vi "SCMP - Externally Triggered Image Acquisition - v4.vi"(0 "FPS":dbl=10.0 format="%.1g", 1 "LCVR Voltages":dbl[][](array[numeric]), 2 "Mod/Seq":bool, 5 "Cycles":i32=1 min=1 max=30 step=1, 7 "Save to FITS?":bool=TRUE, 9 "Headers In":T12[](array[typedef])=[{"Wavelength (nm)"=530.15, "Exposure (s)"=0.05, "Tuning Delay (ms)"=1000.0, "Beam Type (-1/1)"=1.0, "Tuning Voltages"=[1.111, 2.222, 3.333, 4.444], "Observer"="observer", "Light Shapping Diffuser"=enum."In Beam", "Comment"="", "Data Type"=9, "Mod Cycles"=0, "SCD Calibration Optics"=enum."1 - Polarizer @0, I+Q", "SCD Emission Line Filter"=enum."1-557.6nm", "Cookbook"="", "COMP-S Calibration Wheel"=enum."Dark", "COMP-S Andover Filter Wheel"=enum."530.3nm/HWB 0.34nm (Fe XIV)", "FOV Rotation (deg)"=66.0, "Objective Lens Position (mm)"=0.0, "Occulter size"=0.0, "Time End"=timestamp(3382374145.421875 s since 1904-01-01), "Acc Exposure (s)"=0.0, "Time Stamp Array"=[], "Camera Serial Number"=[], "Camera Temp"=[], "Camera PI (mm)"=[], "Time Start"=timestamp(3382374145.421875 s since 1904-01-01), "Peripherals"={"ILX controler"=FALSE, "Zone temperatures"=FALSE, "Andor"=FALSE, "Andor 2"=FALSE, "PI Stages"=FALSE, "AISAS mechanisms"=FALSE, "AISAS Mech.lvclass"=refnum, "Zone temp ref"=variant, "FWs"=FALSE}, "FITS paths"=[], "Cameras"=enum."Andor", "load preset cbk"=FALSE, "periodic check count"=0, "COMP-S Calibration Wheel 2"=enum."Dark", "Calib"=enum."Dark", "Abso Aperture"=40.0, "Nominal Aperture"=196.0}] {"Nominal Aperture" format="%.1f"; "Abso Aperture" format="%.1f"; "Camera PI (mm)" format="%_3g"; "Acc Exposure (s)" format="%^.3g"; "Occulter size" format="%.2f"; "Objective Lens Position (mm)" min=70.0 max=152.0 format="%.2f"; "FOV Rotation (deg)" format="%.1f"; "Data Type" items=["LIVE", "DARK", "FLAT", "CALI", "OBSE", "ABSO", "AURE", "TARG", "OBJE", "HOLE", "OREX", "THRO", "CHIP"]; "Exposure (s)" format="%^.3g"; "Wavelength (nm)" format="%_6g"}, 11 "error in":errorcluster, 12 "Andor Neo":T13[](array[typedef]) {"Exposure (s)" format="%^.3g"; "Time at Synch" format="%<%H:%M:%S>T"; "Interframe Time" format="%#_3g"; "Frame Readout Time" format="%_3g"; "Row Readout Time" format="%_3g"}) -> (3 "FITS Path Out":path, 6 "Image":u32[][](array[numeric]), 8 "Camera R Image":u32[][](graph), 10 "Headers Out":T2[](array[typedef]) {"Nominal Aperture" format="%.1f"; "Abso Aperture" format="%.1f"; "Camera PI (mm)" format="%_3g"; "Acc Exposure (s)" format="%^.3g"; "Occulter size" format="%.2f"; "Objective Lens Position (mm)" min=70.0 max=152.0 format="%.2f"; "FOV Rotation (deg)" format="%.1f"; "Exposure (s)" format="%^.3g"; "Wavelength (nm)" format="%_6g"}, 13 "FITS Path Out 2":path, 14 "Break":bool, 15 "error out":errorcluster)   [LabVIEW 2014]
doc: "The LL Sequence VI acquires a sequence of images and displays them in an array of image controls using the low-level acquisition VIs. A sequence is appropriate for applications that process multiple images. You can configure a sequence to acquire every frame or to skip a variable number of frames between each image.\n\nTop Level Code Overview\n1) Initialize Camera (Global Shutter, High Well, Low Noise, exposure time, etc.)\n2) Create a buffer set equal in size to the # of trigger pulses (e.g. 100) which is the same as the # of expected images \n3) Start the camera acquisition THEN start the DAQmx task (use merge error cluster to gurantee this)"
uses:
  Camera/Andor Neo Info.ctl
  Controls/run cbk timeout.ctl
  <vilib>/Waveform/WDTOps.llb/WDT Waveform Duration DBL.vi
  <vilib>/DAQmx/write.llb/DAQmx Write (Analog 1D Wfm NChan NSamp).vi
  <vilib>/DAQmx/create/channels.llb/DAQmx Create Channel (AO-Voltage-Basic).vi
  <vilib>/DAQmx/configure/timing.llb/DAQmx Timing (Use Waveform).vi
  Controls/Global demo.vi
  Controls/beaning.ctl
  Controls/SCD - Calibration Optics Filter Wheel.ctl
  AISAS/Controls/Diffuser.ctl
  Controls/SCD - FITS Cluster.ctl
  Controls/SCD - EDT - Emission Line Filter Wheel.ctl
  Controls/CoMP-S Controls/Polarization Optics Filter Wheel.ctl
  Controls/CoMP-S Controls/Emission Line Filter Wheel.ctl
  AISAS/Controls/focus.ctl
  AISAS/Mech/AISAS Mech.lvclass
  Controls/peripherals.ctl
  Controls/Cameras select.ctl
  Controls/FITS Data type.ctl
panel:
  out "error dequeue RAM":errorcluster
  out "mod cycles *4":i32=1
  out "error cam dequeue & queue RAM":errorcluster
  out "error dequeue 2":errorcluster
  in  "count 2":i32
  in  "Tab Control":T1(tab)
  out "Camera T Image":u32[][](graph)
  out "# elements in RAM queue":i32
  out "Image Acq (s)":dbl(slide)=4151.832132564842
  out "Image display & SSD Saving":i32(slide) scale=0.0..1.0
  in  "user break":bool
  out "Camera T Image wide":u32[][](graph)
  out "# images to acquire":i32
  out "Image Acquisition Started":bool
  out "PixelData [U16]":u16[](array[numeric])
  out "ByteData [U8]":u8[](array[numeric])
  in  "image pointers":u64[](array[numeric])
  in  "imageNo":i32
  in  "count":i32
  out "# wavelengths":i32=1
  out "Exposure Get (s)":dbl=0.09 format="%_3p"
  out "# elements in queue":i32
  out "Image Cam":u32[][](graph)
  out "# buffer":i32
  in  "image pointers 2":u64[](array[numeric])
  in  "imageNo 2":i32
  out "# elements in queue 2":i32
  out "# buffer 2":i32
  out "Image transfering":u32(slide) scale=0.0..4.0
  out "Acquisition Estimate (s)":dbl format="%0.2f"
  out "Image Acq":i32(slide) scale=0.0..4.0
  out "Time Start":timestamp=timestamp(3382374145.421875 s since 1904-01-01) format="%<%H:%M:%S%3u\n%x>T"
  out "Time stamp arr":timestamp[](array[timestamp]) format="%<%H:%M:%S%3u>T"
  out "COMP Waveforms":waveform(dbl)[](graph)
  out "SCD Waveforms":waveform(dbl)[](graph)
  out "Time stamp arr 2":timestamp[](array[timestamp]) format="%<%H:%M:%S%3u>T"
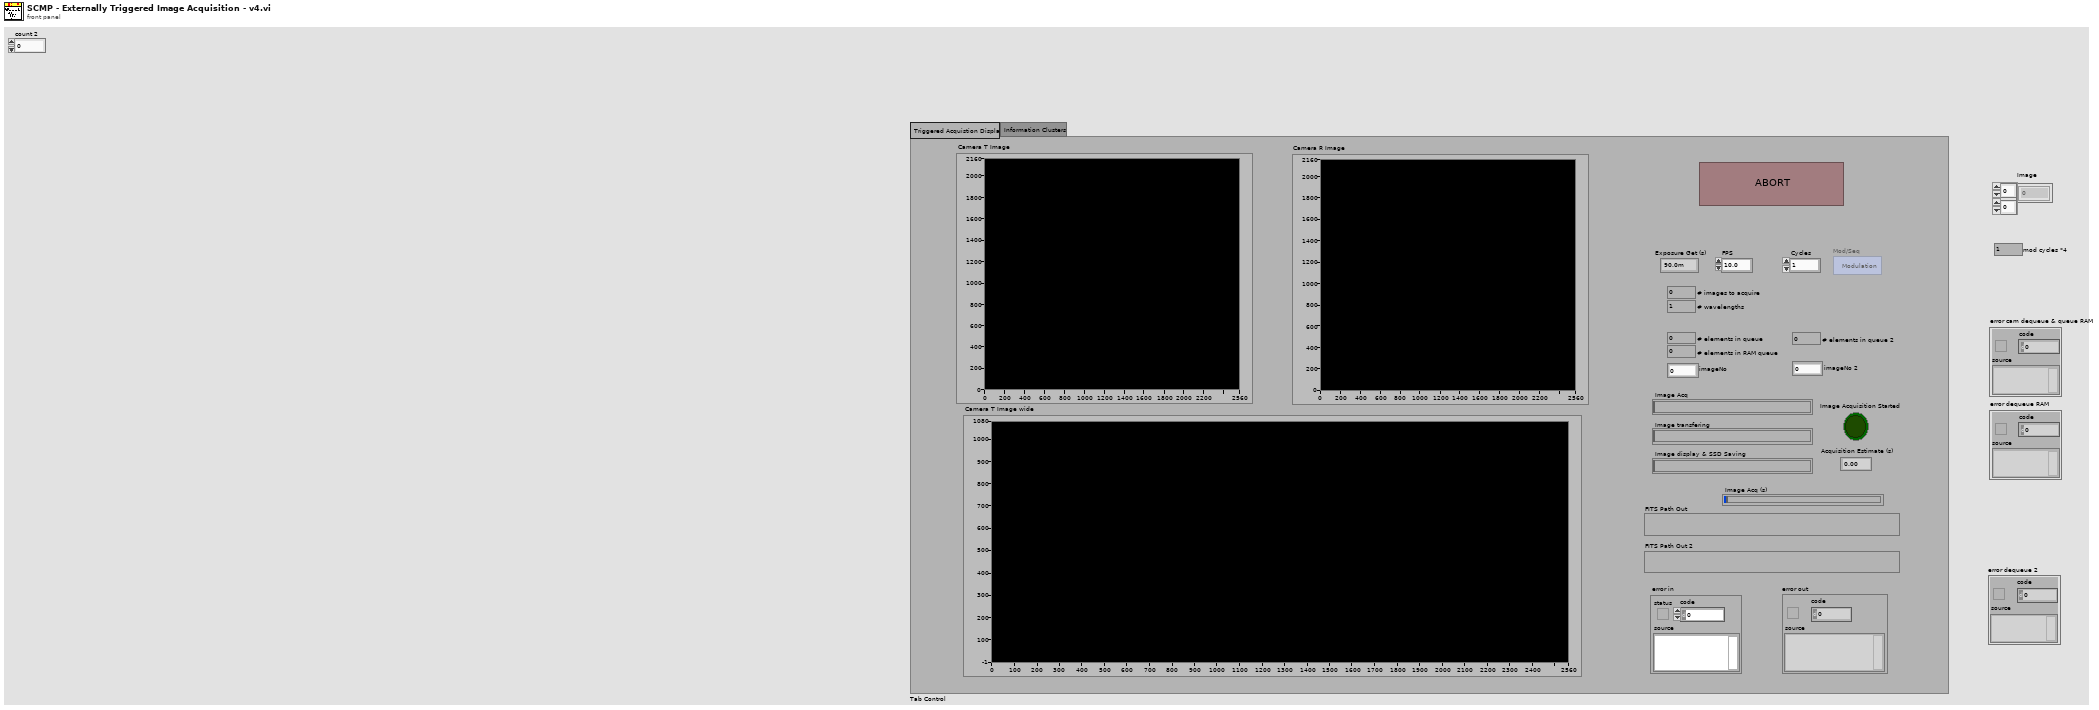
[diagram p1: front panel]
types:
  T1 = enum32{"Triggered Acquistion Display", "Information Clusters"}
  T2 = typedef "SCD - FITS Cluster.ctl" = cluster{"Wavelength (nm)":dbl, "Exposure (s)":dbl, "Tuning Delay (ms)":dbl, "Beam Type (-1/1)":dbl, "Tuning Voltages":dbl[], "Observer":string, "Light Shapping Diffuser":T3, "Comment":string, "Data Type":T4, "Mod Cycles":u16, "SCD Calibration Optics":T5, "SCD Emission Line Filter":T6, "Cookbook":string, "COMP-S Calibration Wheel":T7, "COMP-S Andover Filter Wheel":T8, "FOV Rotation (deg)":dbl, "Objective Lens Position (mm)":T9, "Occulter size":dbl, "Time End":timestamp, "Acc Exposure (s)":dbl, "Time Stamp Array":timestamp[], "Camera Serial Number":string[], "Camera Temp":dbl[], "Camera PI (mm)":dbl[], "Time Start":timestamp, "Peripherals":T10, "FITS paths":path[], "Cameras":T11, "load preset cbk":bool, "periodic check count":i32, "COMP-S Calibration Wheel 2":T7, "Calib":enum16{"Dark", "Flat"}, "Abso Aperture":dbl, "Nominal Aperture":dbl, "Pointer IP":string}
  T3 = typedef "Diffuser.ctl" = enum16{"Out of Beam", "In Beam"}
  T4 = typedef "FITS Data type.ctl" = enum16{"LIVE", "DARK", "FLAT", "CALI", "OBSE", "ABSO", "AURE", "TARG", "OBJE", "HOLE", "OREX", "THRO", "CHIP"}
  T5 = typedef "SCD - Calibration Optics Filter Wheel.ctl" = enum16{"1 - Polarizer @0, I+Q", "2 - Polarizer @90, I-Q", "3 - Polarizer @45, I+U", "4 - Polarizer @135, I-U", "5 - Polarizer @0, Retarder @45, I+V", "6 - Polarizer @0, Retarder @135, I-V", "7 - Dark", "8 - Clear", "9 - N/A"}
  T6 = typedef "SCD - EDT - Emission Line Filter Wheel.ctl" = enum16{"1-557.6nm", "2-587.6nm", "3-589.6nm", "4-630.2nm", "5-656.4nm", "6-849.8nm", "7-854.2nm", "8-866.2nm", "9-1083.0nm"}
  T7 = typedef "Polarization Optics Filter Wheel.ctl" = enum16{"Dark", "Clear", "Exchange Lens", "Polarizer @0, I+Q", "Polarizer @90, I-Q", "Polarizer @45, I+U", "Polarizer @135, I-U", "Polarizer @0, Retarder @45, I+V", "Polarizer @0, Retarder @135, I-V"}
  T8 = typedef "Emission Line Filter Wheel.ctl" = enum16{"530.3nm/HWB 0.34nm (Fe XIV)", "587.6nm/HBW 0.44nm (He I D3)", "637.5nm/HBW 0.53nm (Fe X)", "656.3nm/HBW 0.57nm (H-Alpha)", "789.2nm/HBW 0.85nm (Fe XI)", "854.2nm/HBW 1.01nm (Ca I)", "1074.7nm/HBW 2.34nm (Fe XIII)", "1079.8nm/HBW 1.64nm (Fe XIII)", "1083.0nm/HBW 1.66nm (He I)"}
  T9 = typedef "focus.ctl" = dbl
  T10 = typedef "peripherals.ctl" = cluster{"ILX controler":bool, "Zone temperatures":bool, "Andor":bool, "Andor 2":bool, "PI Stages":bool, "AISAS mechanisms":bool, "AISAS Mech.lvclass":refnum<class "AISAS Mech.lvclass">, "Zone temp ref":variant, "FWs":bool}
  T11 = typedef "Cameras select.ctl" = enum16{"Andor", "GDR"}
  T12 = typedef "SCD - FITS Cluster.ctl" = cluster{"Wavelength (nm)":dbl, "Exposure (s)":dbl, "Tuning Delay (ms)":dbl, "Beam Type (-1/1)":dbl, "Tuning Voltages":dbl[], "Observer":string, "Light Shapping Diffuser":T3, "Comment":string, "Data Type":u16, "Mod Cycles":u16, "SCD Calibration Optics":T5, "SCD Emission Line Filter":T6, "Cookbook":string, "COMP-S Calibration Wheel":T7, "COMP-S Andover Filter Wheel":T8, "FOV Rotation (deg)":dbl, "Objective Lens Position (mm)":T9, "Occulter size":dbl, "Time End":timestamp, "Acc Exposure (s)":dbl, "Time Stamp Array":timestamp[], "Camera Serial Number":string[], "Camera Temp":dbl[], "Camera PI (mm)":dbl[], "Time Start":timestamp, "Peripherals":T10, "FITS paths":path[], "Cameras":T11, "load preset cbk":bool, "periodic check count":i32, "COMP-S Calibration Wheel 2":T7, "Calib":enum16{"Dark", "Flat"}, "Abso Aperture":dbl, "Nominal Aperture":dbl}
  T13 = typedef "Andor Neo Info.ctl" = cluster{"Handle":i32, "Pixel Encoding":string, "AOI Width":i32, "AOI Height":i32, "AOI Stride":i32, "Row Readout Time":dbl, "Frame Readout Time":dbl, "Interframe Time":dbl, "Semaphore":T14, "SerialNumber":string, "Camera Model":string, "Controller ID":string, "Firmware Version":string, "Shutter":string, "BDiv":u8, "Time at Synch":timestamp, "Idx":i32, "PreAmp":string, "Binning":T15, "PixelReadoutRate":string, "Exposure (s)":dbl, "Image Bytes":i64, "Image Pixels":i64, "SpuriousNoiseFilter":bool, "Overlap":bool, "CycleMode":string}
  T14 = typedef "Semaphore RefNum" = refnum<k1>
  T15 = typedef "beaning.ctl" = enum16{"1x1", "2x2", "3x3", "4x4", "8x8"}
  T16 = enum8{"Enabled", "Disabled", "Disabled and Grayed Out"}
  T17 = typedef "run cbk timeout.ctl" = i32
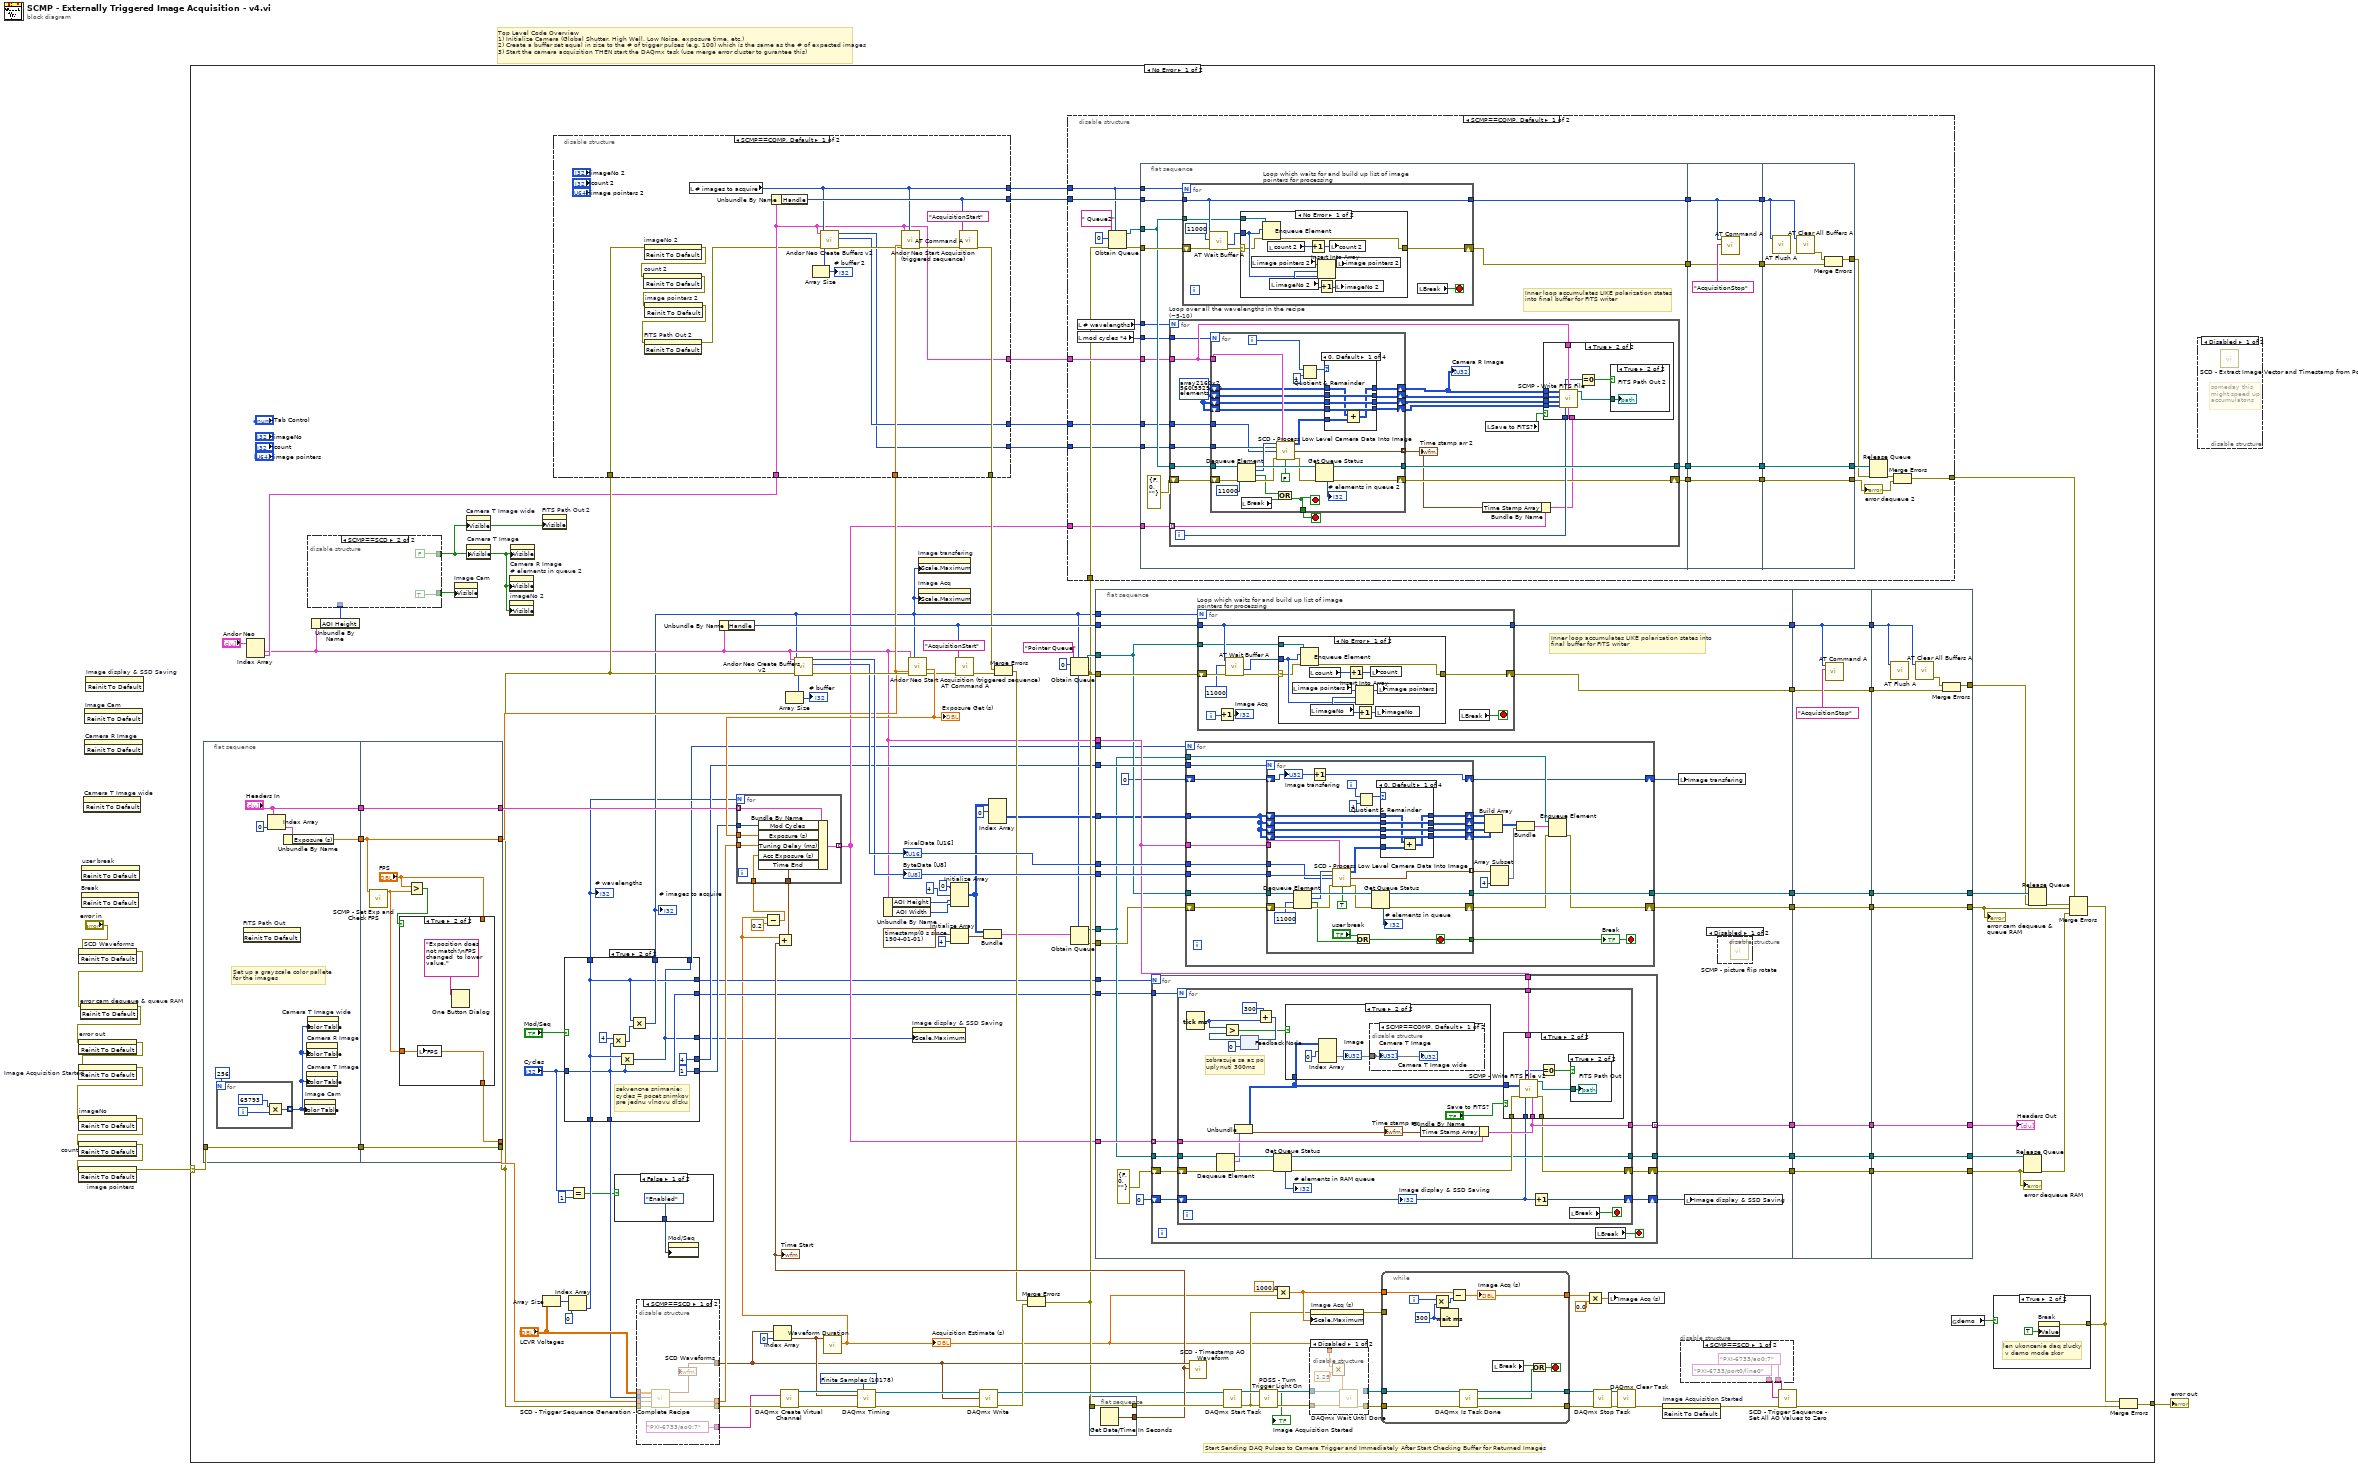
[diagram p0: block diagram]
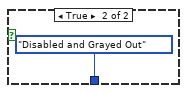
[diagram p3: hidden frame]
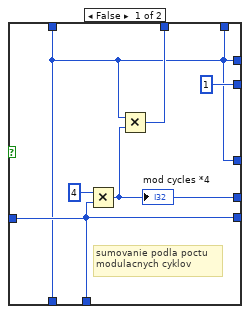
[diagram p6: hidden frame]
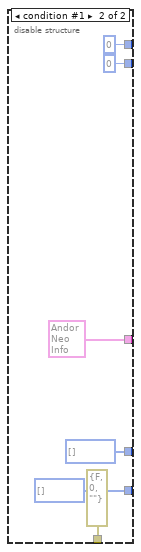
[diagram p7: hidden frame]
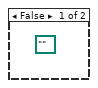
[diagram p8: hidden frame]
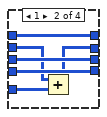
[diagram p10: hidden frame]
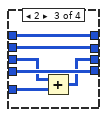
[diagram p11: hidden frame]
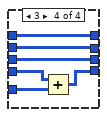
[diagram p12: hidden frame]
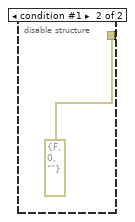
[diagram p14: hidden frame]
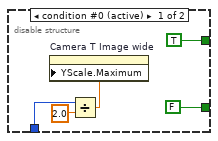
[diagram p16: hidden frame]
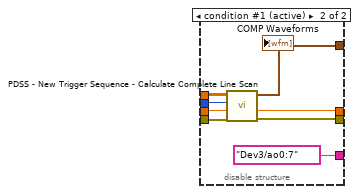
[diagram p17: hidden frame]
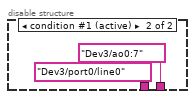
[diagram p18: hidden frame]
diagram:
  # "Top Level Code Overview\n1) Initialize Camera (Global Shutter, High Well, Low Noise, exposure time, etc.)\n2) Create a buffer set equal in size to the # of trigger pulses (e.g. 100) which is the same as the # of expected images \n3) Start the camera acquisition THEN start the DAQmx task (use merge error cluster to gurantee this)"
  n1 = invoke on="SCD Waveforms" class="WFGraph (strict)" method="Reinit To Default"(error in="error in") -> (error out=w3:errorcluster)  [unwired: 2 in, 2 out]
  n2 = invoke on="error cam dequeue & queue RAM" class="Clust (strict)" method="Reinit To Default"(error in=w3) -> (error out=w2:errorcluster)  [unwired: 2 in, 2 out]
  n3 = invoke on="error out" class="Clust (strict)" method="Reinit To Default"(error in=w2) -> (error out=w8:errorcluster)  [unwired: 2 in, 2 out]
  n4 = invoke on="Image Acquisition Started" class="Bool (strict)" method="Reinit To Default"(error in=w8) -> (error out=w4:errorcluster)  [unwired: 2 in, 2 out]
  n5 = invoke on="imageNo" class="DigNum (strict)" method="Reinit To Default"(error in=w4) -> (error out=w7:errorcluster)  [unwired: 2 in, 2 out]
  n6 = invoke on="count" class="DigNum (strict)" method="Reinit To Default"(error in=w7) -> (error out=w6:errorcluster)  [unwired: 2 in, 2 out]
  n7 = invoke on="image pointers" class="Arr (strict)" method="Reinit To Default"(error in=w6) -> (error out=w5:errorcluster)  [unwired: 2 in, 2 out]
  n8 = invoke on="Break" class="Bool (strict)" method="Reinit To Default"() -> ()  [unwired: 3 in, 3 out]
  n9 = invoke on="user break" class="Bool (strict)" method="Reinit To Default"() -> ()  [unwired: 3 in, 3 out]
  n10 = invoke on="Camera T Image wide" class="IntGraph (strict)" method="Reinit To Default"() -> ()  [unwired: 3 in, 3 out]
  n11 = invoke on="Image Cam" class="IntGraph (strict)" method="Reinit To Default"() -> ()  [unwired: 3 in, 3 out]
  n12 = invoke on="Camera R Image" class="IntGraph (strict)" method="Reinit To Default"() -> ()  [unwired: 3 in, 3 out]
  n13 = invoke on="Image display & SSD Saving" class="Slide (strict)" method="Reinit To Default"() -> ()  [unwired: 3 in, 3 out]
  n14 = case shown="No Error" w5 {
    selector: w5 -> [w92 w610]
    tunnel: [w120 w610] -> w9
    frame No Error {
      w143 = 10178 items=["Finite Samples"=10178, "Continuous Samples"=10123] ("sample mode")
      # "Start Sending DAQ Pulses to Camera Trigger and Immediately After Start Checking Buffer for Returned Images"
      n15 = flat-sequence {
        tunnel: w92 -> [w365]
        tunnel: [w365] -> w84
        tunnel: ["Headers In"] -> w82
        tunnel: [w361] -> w81
        tunnel: [w376] -> w63
        tunnel: w84 -> [w376]
        tunnel: [w375] -> w83
        tunnel: w82 -> [w375]
        tunnel: [w370] -> w73
        tunnel: w81 -> [w370]
        tunnel: [w373] -> w80
        frame #0 {
          # "Set up a grayscale color pallete for the images"
          n16 = for {
            N: 256 -> [_]
            tunnel: [w368] -> w360 mode=indexing
            i -> [w369]
            n17 = Multiply(x=65793, y=w369) -> (x*y=w368:i32)
          }
          n18 = invoke on="FITS Path Out" class="Path" method="Reinit To Default"() -> ()  [unwired: 3 in, 3 out]
          n19 = Index Array(array="Headers In", index=0) -> (element=w363:T12)
          n20 = Unbundle By Name(w363) -> ("Exposure (s)"=w361:dbl)
          n21 = property on="Image Cam" class="IntGraph (strict)"("Color Table"=w360) -> ()  [unwired: 2 in, 2 out]
          n22 = property on="Camera R Image" class="IntGraph (strict)"("Color Table"=w360) -> ()  [unwired: 2 in, 2 out]
          n23 = property on="Camera T Image" class="IntGraph (strict)"("Color Table"=w360) -> ()  [unwired: 2 in, 2 out]
          n24 = property on="Camera T Image wide" class="IntGraph (strict)"("Color Table"=w360) -> ()  [unwired: 2 in, 2 out]
        }
        frame #1 {
          n25 = call "SCMP - Set Exp and Check FPS.vi"("Exposure [s]"=w370) -> ("FPS"=w371:dbl)  [unwired: 9 in, 1 out]
          n26 = Greater?(x="FPS", y=w371) -> (0:w374:bool)
          n27 = case shown="True" w374 {
            tunnel: [w377 w378] -> w373
            tunnel: "FPS" -> [w377 _]
            tunnel: w371 -> [_ w378]
            frame False {
            }
            frame True {
              n28 = local write "FPS"(w378) -> ()
              n29 = One Button Dialog(message="Exposition does not match!\nFPS changed  to lower value.") -> ()  [unwired: 1 in, 1 out]
            }
          }
        }
      }
      n30 = Index Array(array="Andor Neo") -> (element #1=w55:T13, element #2=w60:T13)  [unwired: 2 in]
      n31 = Unbundle By Name(w55) -> ("AOI Height"=w99:i32)
      n32 = disable-structure shown="SCMP==SCD" {
        disable-tunnel: w99 -> [w383 _]
        disable-tunnel: [TRUE ("Visible") FALSE ("Visible")] -> w10
        disable-tunnel: [FALSE ("Visible") TRUE ("Visible")] -> w98
        frame condition #0 (active) {
          n33 = Divide(x=w383, y=2.0) -> (x/y=w384:dbl)
          n34 = property on="Camera T Image wide" class="IntGraph (strict)"("YScale.Maximum"=w384) -> ()  [unwired: 2 in, 2 out]
        }
        frame condition #1 {
        }
      }
      n35 = property on="Image Cam" class="IntGraph (strict)"("Visible"=w98) -> ()  [unwired: 2 in, 2 out]
      n36 = property on="Camera T Image wide" class="IntGraph (strict)"("Visible"=w10) -> ()  [unwired: 2 in, 2 out]
      n37 = property on="Camera T Image" class="IntGraph (strict)"("Visible"=w10) -> ()  [unwired: 2 in, 2 out]
      n38 = property on="# elements in queue 2" class="DigNum (strict)"("Visible"=w10) -> ()  [unwired: 2 in, 2 out]
      n39 = property on="imageNo 2" class="DigNum (strict)"("Visible"=w10) -> ()  [unwired: 2 in, 2 out]
      n40 = property on="Camera R Image" class="IntGraph (strict)"("Visible"=w10) -> ()  [unwired: 2 in, 2 out]
      n41 = property on="FITS Path Out 2" class="Path"("Visible"=w10) -> ()  [unwired: 2 in, 2 out]
      n42 = Array Size(array="LCVR Voltages") -> (size(s)=w129:i32[])
      n43 = disable-structure shown="SCMP==COMP, Default" {
        disable-tunnel: w73 -> [w198 _]
        disable-tunnel: [w197 errorcluster {"status"=FALSE, "code"=0, "source"=""} ("error out")] -> w70
        disable-tunnel: [w191 0 ("Handle")] -> w67
        disable-tunnel: [w190 i64[] [] ("PixelData")] -> w66
        disable-tunnel: [w189 u8[] [] ("ByteData")] -> w65
        disable-tunnel: [w188 0 ("# images to acquire")] -> w64
        disable-tunnel: w63 -> [w184 _]
        disable-tunnel: [w187 T13 {"Handle"=0, "Pixel Encoding"="", "AOI Width"=0, "AOI Height"=0, "AOI Stride"=0, "Row Readout Time"=0.0, "Frame Readout Time"=0.0, "Interframe Time"=0.0, "Semaphore"=refnum, "SerialNumber"="", "Camera Model"="", "Controller ID"="", "Firmware Version"="", "Shutter"="Global", "BDiv"=1, "Time at Synch"=timestamp(3029526000.379448 s since 1904-01-01), "Idx"=0, "PreAmp"="", "Binning"=enum."1x1", "PixelReadoutRate"="", "Exposure (s)"=0.05, "Image Bytes"=0, "Image Pixels"=0, "SpuriousNoiseFilter"=FALSE, "Overlap"=FALSE, "CycleMode"=""} ("Neo Info")] -> w61
        disable-tunnel: w60 -> [w187 _]
        frame condition #0 (active) {
          n44 = invoke on="imageNo 2" class="DigNum (strict)" method="Reinit To Default"(error in=w184) -> (error out=w186:errorcluster)  [unwired: 2 in, 2 out]
          n45 = invoke on="count 2" class="DigNum (strict)" method="Reinit To Default"(error in=w186) -> (error out=w185:errorcluster)  [unwired: 2 in, 2 out]
          n46 = invoke on="image pointers 2" class="Arr (strict)" method="Reinit To Default"(error in=w185) -> (error out=w183:errorcluster)  [unwired: 2 in, 2 out]
          n47 = invoke on="FITS Path Out 2" class="Path" method="Reinit To Default"(error in=w183) -> (error out=w182:errorcluster)  [unwired: 2 in, 2 out]
          n48 = local read "# images to acquire"() -> (w188:i32)
          n49 = Unbundle By Name(w187) -> ("Handle"=w191:i32)
          n50 = call "Andor Neo Create Buffers v2.vi"("error in"=w182, "Number of Images"=w188, "Camera Info"=w187) -> ("error out"=w195:errorcluster, "PixelData"=w190:i64[], "ByteData"=w189:u8[], "# of Andor buffers"=w193:i32)  [unwired: 4 in, 1 out]
          n51 = Array Size(array=w193) -> (size(s)=→"# buffer 2":i32)
          n52 = call "Andor Neo Start Acquisition (triggered sequence).vi"("Exposure Set (s)"=w198, "error in"=w195, "Frames"=w188, "Camera Info"=w187) -> ("error out"=w194:errorcluster)  [unwired: 6 in, 1 out]
          n53 = call <userlib>:"AT Command A.vi"("error in (no error)"=w194, "Feature"="AcquisitionStart" ("Command"), "Handle"=w191) -> ("error out"=w197:errorcluster)  [unwired: 7 in, 1 out]
        }
        frame condition #1 {
        }
      }
      n54 = Index Array(array=w129, index=0) -> (element=w30:i32)
      n55 = case shown="True" "Mod/Seq" {
        tunnel: [w160 4] -> w62
        tunnel: [w158 w167] -> w34
        tunnel: [w156 w164] -> w27
        tunnel: [w156 w164] -> w29
        tunnel: w30 -> [w156 w164]
        tunnel: [w159 1 ("Cycles")] -> w32
        tunnel: [w159 w163] -> w31
        tunnel: "Cycles" -> [w159 w163]
        tunnel: [w156 w162] -> w28
        tunnel: [1 ("value") w163] -> w26
        tunnel: [w156 w162] -> w25
        frame False {
          # "sumovanie podla poctu\nmodulacnych cyklov"
          n56 = Multiply(x=4 ("value"), y=w159) -> (x*y=w160:i32)
          "mod cycles *4" <- w160
          n57 = Multiply(x=w156, y=w160) -> (x*y=w158:i32)
        }
        frame True {
          # "sekvencne snimanie:\ncycles = pocet snimkov\npre jednu vlnovu dlzku"
          n58 = Multiply(x=4 ("value"), y=w163) -> (x*y=w168:i32)
          n59 = Multiply(x=w164, y=w163) -> (x*y=w162:i32)
          n60 = Multiply(x=w164, y=w168) -> (x*y=w167:i32)
        }
      }
      "# wavelengths" <- w29
      "# images to acquire" <- w34
      n61 = Equal?(x="Cycles", y=1) -> (x = y?=w12:bool)
      n62 = case shown="False" w12 {
        tunnel: [T16."Enabled" ("Disabled") T16."Disabled and Grayed Out" ("Disabled")] -> w11
        frame False {
        }
        frame True {
        }
      }
      n63 = disable-structure shown="SCMP==SCD" {
        disable-tunnel: [w394 w398] -> w136
        disable-tunnel: "LCVR Voltages" -> [w393 w402]
        disable-tunnel: [w388 w396] -> w104
        disable-tunnel: w80 -> [w392 w400]
        disable-tunnel: w63 -> [w391 w399]
        disable-tunnel: [w390 w397] -> w105
        disable-tunnel: w31 -> [w389 w401]
        disable-tunnel: [tag "PXI-6733/ao0:7" ("physical channels") tag "Dev3/ao0:7" ("physical channels")] -> w78
        frame condition #0 {
          n64 = call "SCD - Trigger Sequence Generation - Complete Recipe.vi"("error in"=w391, "FPS"=w392, "Modulation Cycles\nAt Each Wavelength"=w389, "LCVR Voltages"=w393) -> ("error out"=w394:errorcluster, "LCVR Relaxtion Time"=w390:dbl, "SCD Waveforms (Graph)"=w388:waveform(dbl)[])  [unwired: 5 in]
          "SCD Waveforms" <- w388
        }
        frame condition #1 (active) {
          n65 = call "PDSS - New Trigger Sequence - Calculate Complete Line Scan.vi"("error in"=w399, "FPS"=w400, "Modulation Cycles\nAt Each Wavelength"=w401, "LCVR Voltages"=w402) -> ("error out"=w398:errorcluster, "LCVR Relaxtion Time"=w397:dbl, "AO Graph"=w396:waveform(dbl)[])  [unwired: 5 in]
          "COMP Waveforms" <- w396
        }
      }
      n66 = property on="Mod/Seq" class="Bool (strict)"("DisabledEnum"=w11) -> ()  [unwired: 2 in, 2 out]
      n67 = Unbundle By Name(w55) -> ("Handle"=w75:i32)
      n68 = Index Array(array=w104, index=0) -> (element=w133:waveform(dbl))
      n69 = call-poly <vilib>:"DAQmx Create Virtual Channel.vi"("physical channels"=w78, "error in"=w136) -> ("task out"=w141:refnum<k21>, "error out"=w142:errorcluster)  [unwired: 12 in]
      n70 = call "Andor Neo Create Buffers v2.vi"("error in"=w63, "Number of Images"=w34, "Camera Info"=w55) -> ("error out"=w119:errorcluster, "PixelData"=w115:i64[], "ByteData"=w114:u8[], "# of Andor buffers"=w91:i32)  [unwired: 4 in, 1 out]
      "ByteData [U8]" <- w114
      "PixelData [U16]" <- w115
      n71 = Array Size(array=w91) -> (size(s)=→"# buffer":i32)
      n72 = call-poly <vilib>:"Waveform Duration.vi"("waveform in"=w133) -> ("duration"=w22:dbl)  [unwired: 8 in, 2 out]
      "Acquisition Estimate (s)" <- w22
      n73 = Subtract(x=w22, y=0.2) -> (x-y=w93:dbl)
      n74 = Add(x=w22, y=w79) -> (x+y=w97:timestamp)
      n75 = call-poly <vilib>:"DAQmx Timing.vi"("task/channels in"=w141, "sample mode"=w143, "waveform"=w133, "error in"=w142) -> ("task out"=w134:refnum<k21>, "error out"=w135:errorcluster)  [unwired: 10 in]
      n76 = Unbundle By Name(w55) -> ("AOI Height"=w37:i32, "AOI Width"=w36:i32)
      n77 = call "Andor Neo Start Acquisition (triggered sequence).vi"("Exposure Set (s)"=w73, "error in"=w119, "Frames"=w34, "Camera Info"=w55) -> ("error out"=w95:errorcluster, "Exposure Get (s)"=w96:dbl)  [unwired: 6 in]
      "Exposure Get (s)" <- w96
      n78 = for {
        N: w29 -> [_]
        tunnel: [w413] -> w69 mode=indexing
        tunnel: w96 -> [w412]
        tunnel: w83 -> [w411] mode=indexing
        tunnel: w105 -> [w410]
        tunnel: w32 -> [w409]
        tunnel: w93 -> [w408]
        tunnel: w97 -> [w407]
        n79 = Bundle By Name(cluster=w411, "Mod Cycles"=w409, "Exposure (s)"=w412, "Tuning Delay (ms)"=w410, "Acc Exposure (s)"=w408, "Time End"=w407) -> (w413:T12)
      }
      n80 = property on="Image display & SSD Saving" class="Slide (strict)"("Scale.Maximum"=w25) -> ()  [unwired: 2 in, 2 out]
      n81 = property on="Image transfering" class="Slide (strict)"("Scale.Maximum"=w34) -> ()  [unwired: 2 in, 2 out]
      n82 = property on="Image Acq" class="Slide (strict)"("Scale.Maximum"=w34) -> ()  [unwired: 2 in, 2 out]
      n83 = Initialize Array(u32 0, 4 ("dimension size"), w37, w36) -> (w40:u32[][][])
      n84 = Initialize Array(timestamp(0 s since 1904-01-01) ("Timestamp"), 4 ("dimension size")) -> (w49:timestamp[])
      n85 = call <userlib>:"AT Command A.vi"("error in (no error)"=w95, "Feature"="AcquisitionStart" ("Command"), "Handle"=w75) -> ("error out"=w118:errorcluster)  [unwired: 7 in, 1 out]
      n86 = call-poly <vilib>:"DAQmx Write.vi"("task/channels in"=w134, "data"=w104, "error in"=w135) -> ("task out"=w74:refnum<k21>, "error out"=w122:errorcluster)  [unwired: 10 in, 1 out]
      n87 = Bundle(w40, w49) -> (w35:cluster{u32[][][], timestamp[]})  [unwired: 1 in]
      n88 = Index Array(array=w40, index (dim 0)=0 ("disabled index (col)")) -> (element=w39:u32[][])  [unwired: 2 in]
      n89 = Merge Errors(w70, w118) -> (w71:errorcluster)
      n90 = Merge Errors(w71, w122) -> (w72:errorcluster)
      n91 = disable-structure shown="SCMP==COMP, Default" {
        disable-tunnel: w61 -> [w222 _]
        disable-tunnel: w72 -> [w221 _]
        disable-tunnel: w69 -> [w220 _]
        disable-tunnel: [w219 errorcluster {"status"=FALSE, "code"=0, "source"=""} ("error IO")] -> w68
        disable-tunnel: w67 -> [w216 _]
        disable-tunnel: w66 -> [w215 _]
        disable-tunnel: w65 -> [w214 _]
        disable-tunnel: w64 -> [w211 _]
        frame condition #0 (active) {
          n92 = local read "# wavelengths"() -> (w210:i32)
          n93 = local read "mod cycles *4"() -> (w205:i32)
          n94 = Obtain Queue(max queue size (-1, unlimited)=w211, name (unnamed)=" Queue2", element data type=u64 0 ("Output buffer"), error in (no error)=w221) -> (queue out=w213:refnum<queue>, error out=w212:errorcluster)  [unwired: 1 in, 1 out]
          n95 = flat-sequence {
            tunnel: w212 -> [w245]
            tunnel: w216 -> [w244]
            tunnel: [w243] -> w230
            tunnel: [w234] -> w229
            tunnel: w222 -> [w238]
            tunnel: w215 -> [w239]
            tunnel: w214 -> [w241]
            tunnel: w213 -> [w242]
            tunnel: [w240] -> w228
            tunnel: w205 -> [w236]
            tunnel: [w237] -> w227
            tunnel: w211 -> [w233]
            tunnel: w220 -> [w232]
            tunnel: w210 -> [w231]
            tunnel: w230 -> [w349]
            tunnel: w229 -> [w348]
            tunnel: w228 -> [w351]
            tunnel: w227 -> [w350]
            tunnel: [w349] -> w226
            tunnel: [w351] -> w225
            tunnel: [w350] -> w224
            tunnel: [w348] -> w223
            tunnel: [w358] -> w207
            tunnel: [w357] -> w206
            tunnel: w226 -> [w355]
            tunnel: w225 -> [w353]
            tunnel: w224 -> [w358]
            tunnel: w223 -> [w356]
            tunnel: [w353] -> w208
            frame #0 {
              # "Inner loop accumulates LIKE polarization states into final buffer for FITS writer"
              n96 = for "Loop over all the wavelengths in the recipe (~5-10)" {
                N: w231 -> [_]
                tunnel: w242 -> [w264]
                tunnel: w241 -> [w263]
                tunnel: [w262] -> w240
                tunnel: w239 -> [w261]
                tunnel: w238 -> [w259]
                tunnel: w236 -> [w258]
                shift-right: [w256] -> w237
                shift-left: errorcluster {"status"=FALSE, "code"=0, "source"=""} ("error out") -> [w255]
                tunnel: w232 -> [w251] mode=indexing
                i -> [w257]
                stop <- w254 stop-if-true
                w260 = u32[][] array2160x2560[5529600 elements] ("2560x2160 Initialized Array")
                n97 = for {
                  N: w258 -> [_]
                  tunnel: w264 -> [w304]
                  tunnel: w263 -> [w301]
                  tunnel: [w287] -> w262
                  tunnel: w261 -> [w300]
                  tunnel: w259 -> [w299]
                  shift-right: [w292] -> w249
                  shift-left: w260 -> [w293]
                  shift-right: [w291] -> w248
                  shift-left: w260 -> [w294]
                  shift-right: [w290] -> w247
                  shift-left: w260 -> [w295]
                  shift-right: [w289] -> w246
                  shift-left: w260 -> [w296]
                  shift-right: [w282] -> w256
                  shift-left: w255 -> [w280]
                  tunnel: [w277] -> w254
                  tunnel: [w279] -> w252 mode=indexing
                  i -> [w281]
                  stop <- w277 stop-if-true
                  n98 = Dequeue Element(queue=w304, timeout in ms (-1)=11000, error in (no error)=w280) -> (queue out=w303:refnum<queue>, element=w302:u64, timed out?=w276:bool, error out=w284:errorcluster)
                  n99 = local read "Break"() -> (w275:bool)
                  n100 = Or(x=w276, y=w275) -> (x .or. y?=w277:bool)
                  n101 = call "SCD - Process Low Level Camera Data Into Image.vi"("Pointer In"=w302, "Neo Info"=w299, "ByteData (U8)"=w301, "PixelData (U16)"=w300, "error in (no error)"=w284, "scmp demo pic"=FALSE) -> ("Image (I32)"=w288:u32[][], "Timestamp"=w279:timestamp, "error out"=w283:errorcluster)  [unwired: 7 in]
                  n102 = Quotient & Remainder(x=w281, y=4) -> (x-y*floor(x/y)=w297:i32)  [unwired: 1 out]
                  n103 = Get Queue Status(queue=w303, error in (no error)=w283) -> (queue out=w287:refnum<queue>, error out=w282:errorcluster, # elements in queue=→"# elements in queue 2":i32)  [unwired: 1 in, 5 out]
                  n104 = case shown="0, Default" w297 {
                    tunnel: w296 -> [w308 w315 w321 w324]
                    tunnel: w295 -> [w309 w316 w318 w327]
                    tunnel: w294 -> [w310 w312 w322 w328]
                    tunnel: w293 -> [w306 w313 w319 w325]
                    tunnel: [w305 w313 w319 w325] -> w292
                    tunnel: [w310 w311 w322 w328] -> w291
                    tunnel: [w309 w316 w317 w327] -> w290
                    tunnel: [w308 w315 w321 w323] -> w289
                    tunnel: w288 -> [w307 w314 w320 w326]
                    frame 0, Default {
                      n105 = Add(x=w306, y=w307) -> (x+y=w305:u32[][])
                    }
                    frame 1 {
                      n106 = Add(x=w312, y=w314) -> (x+y=w311:u32[][])
                    }
                    frame 2 {
                      n107 = Add(x=w318, y=w320) -> (x+y=w317:u32[][])
                    }
                    frame 3 {
                      n108 = Add(x=w324, y=w326) -> (x+y=w323:u32[][])
                    }
                  }
                }
                "Time stamp arr 2" <- w252
                "Camera R Image" <- w249
                n109 = Bundle By Name(cluster=w251, "Time Stamp Array"=w252) -> (w253:T12)
                n110 = local read "Save to FITS?"() -> (w250:bool)
                n111 = case shown="True" w250 {
                  tunnel: w248 -> [_ w271]
                  tunnel: w247 -> [_ w272]
                  tunnel: w246 -> [_ w273]
                  tunnel: w253 -> [_ w269]
                  tunnel: w249 -> [_ w270]
                  tunnel: w259 -> [_ w268]
                  tunnel: w257 -> [_ w267]
                  frame False {
                    (unwired) path "" ("FITS Path Out")
                  }
                  frame True {
                    n112 = call "SCMP - Write FITS File.vi"("A"=w270, "FITS Header"=w269, "Neo Info"=w268, "B"=w271, "C"=w272, "D"=w273, "Image #"=w267) -> ("FITS Path Out"=w266:path)  [unwired: 6 in, 2 out]
                    n113 = Equal To 0?(x=w267) -> (x = 0?=w265:bool)
                    n114 = case shown="True" w265 {
                      tunnel: w266 -> [_ w274]
                      frame False {
                      }
                      frame True {
                        "FITS Path Out 2" <- w274
                      }
                    }
                  }
                }
              }
              n115 = for "Loop which waits for and build up list of image pointers for processing" {
                N: w233 -> [_]
                tunnel: w244 -> [w333]
                tunnel: [w333] -> w243
                tunnel: w242 -> [w331]
                shift-right: [w330] -> w234
                shift-left: w245 -> [w335]
                stop <- w329 stop-if-true
                n116 = call <userlib>:"AT Wait Buffer A.vi"("error in (no error)"=w335, "Timeout"=u32 11000, "Handle"=w333) -> ("error out"=w332:errorcluster, "Output buffer"=w334:u64)  [unwired: 5 in, 2 out]
                n117 = case shown="No Error" w332 {
                  selector: w332 -> [w338 w347]
                  tunnel: w334 -> [w340 _]
                  tunnel: [w337 w347] -> w330
                  tunnel: w331 -> [w339 _]
                  frame No Error {
                    n118 = local read "image pointers 2"() -> (w344:u64[])
                    n119 = Enqueue Element(queue=w339, element=w340, error in (no error)=w338) -> (error out=w337:errorcluster)  [unwired: 1 in, 2 out]
                    n120 = local read "count 2"() -> (w346:i32)
                    n121 = local read "imageNo 2"() -> (w341:i32)
                    n122 = Increment(x=w346) -> (x+1=w345:i32)
                    n123 = Insert Into Array(array=w344, index=w341, new element=w340) -> (w343:u64[])
                    n124 = Increment(x=w341) -> (x+1=w342:i32)
                    n125 = local write "count 2"(w345) -> ()
                    n126 = local write "imageNo 2"(w342) -> ()
                    n127 = local write "image pointers 2"(w343) -> ()
                  }
                  frame Error {
                  }
                }
                n128 = local read "Break"() -> (w329:bool)
              }
            }
            frame #1 {
              n129 = call <userlib>:"AT Command A.vi"("Feature"="AcquisitionStop" ("Command"), "Handle"=w349) -> ()  [unwired: 8 in, 2 out]
            }
            frame #2 {
              n130 = call <userlib>:"AT Flush A.vi"("Handle"=w355) -> ()  [unwired: 9 in, 2 out]
              n131 = call <userlib>:"AT Clear All Buffers A.vi"("Handle"=w355) -> ("error out"=w354:errorcluster)  [unwired: 9 in, 1 out]
              n132 = Merge Errors(w354, w356) -> (w357:errorcluster)
            }
          }
          n133 = Release Queue(queue=w208, error in (no error)=w206) -> (error out=w209:errorcluster)  [unwired: 1 in, 2 out]
          n134 = Merge Errors(w209, w207) -> (w219:errorcluster)
          "error dequeue 2" <- w207
        }
        frame condition #1 {
        }
      }
      n135 = Obtain Queue(max queue size (-1, unlimited)=w34, name (unnamed)="Pointer Queue", element data type=u64 0 ("Output buffer"), error in (no error)=w72) -> (queue out=w111:refnum<queue>, error out=w112:errorcluster)  [unwired: 1 in, 1 out]
      n136 = Obtain Queue(max queue size (-1, unlimited)=w34, element data type=w35) -> (queue out=w52:refnum<queue>, error out=w53:errorcluster)  [unwired: 3 in, 1 out]
      n137 = flat-sequence {
        tunnel: [w415] -> w117
        tunnel: w72 -> [w415]
        tunnel: [w414] -> w79
        frame #0 {
          n138 = Get Date/Time In Seconds() -> (seconds since 1Jan1904=w414:timestamp)
        }
      }
      n139 = flat-sequence {
        tunnel: w112 -> [w442]
        tunnel: w34 -> [w434]
        tunnel: w75 -> [w441]
        tunnel: [w440] -> w124
        tunnel: [w432] -> w123
        tunnel: w55 -> [w431]
        tunnel: w69 -> [w436]
        tunnel: [w435] -> w116
        tunnel: w115 -> [w437]
        tunnel: w114 -> [w439]
        tunnel: w111 -> [w427]
        tunnel: [w438] -> w109
        tunnel: w62 -> [w433]
        tunnel: [w430] -> w102
        tunnel: w53 -> [w429]
        tunnel: w52 -> [w423]
        tunnel: w27 -> [w418]
        tunnel: [w426] -> w48
        tunnel: [w425] -> w46
        tunnel: w39 -> [w424]
        tunnel: w28 -> [w417]
        tunnel: w26 -> [w416]
        tunnel: w124 -> [w596]
        tunnel: w123 -> [w595]
        tunnel: w116 -> [w599]
        tunnel: w109 -> [w598]
        tunnel: w102 -> [w597]
        tunnel: [w596] -> w89
        tunnel: [w599] -> w88
        tunnel: [w598] -> w87
        tunnel: [w597] -> w86
        tunnel: [w595] -> w85
        tunnel: w48 -> [w594]
        tunnel: [w594] -> w47
        tunnel: w46 -> [w593]
        tunnel: [w593] -> w45
        tunnel: [w607] -> w76
        tunnel: [w608] -> w108
        tunnel: [w609] -> w106
        tunnel: [w606] -> w107
        tunnel: w89 -> [w604]
        tunnel: w88 -> [w609]
        tunnel: w87 -> [w608]
        tunnel: w86 -> [w607]
        tunnel: w85 -> [w605]
        tunnel: w47 -> [w602]
        tunnel: [w602] -> w42
        tunnel: w45 -> [w601]
        tunnel: [w601] -> w44
        frame #0 {
          # "Inner loop accumulates LIKE polarization states into final buffer for FITS writer"
          n140 = for {
            N: w418 -> [_]
            tunnel: w436 -> [w453] mode=indexing
            tunnel: [w452] -> w435 mode=indexing
            tunnel: w431 -> [w451]
            shift-right: [w450] -> w426
            shift-left: errorcluster {"status"=FALSE, "code"=0, "source"=""} ("error out") -> [w449]
            tunnel: w423 -> [w448]
            tunnel: [w447] -> w425
            shift-right: [w446] -> w420
            shift-left: 0 -> [w445]
            tunnel: w416 -> [w444]
            stop <- w443 stop-if-true
            n141 = for {
              N: w444 -> [_]
              tunnel: w451 -> [w475]
              shift-right: [w473] -> w450
              shift-left: w449 -> [w472]
              shift-right: [w456] -> w446
              shift-left: w445 -> [w455]
              tunnel: w453 -> [w477]
              tunnel: [w476] -> w452
              tunnel: w448 -> [w469]
              tunnel: [w467] -> w447
              stop <- w454 stop-if-true
              # "zobrazuje sa az po uplynuti 300ms"
              n142 = Tick Count (ms)() -> (millisecond timer value=w460:u32)
              n143 = Dequeue Element(queue=w469, error in (no error)=w472) -> (queue out=w468:refnum<queue>, element=w464:cluster{u32[][][], timestamp[]}, error out=w471:errorcluster)  [unwired: 1 in, 1 out]
              n144 = Unbundle(w464) -> (w463:u32[][][], w466:timestamp[])
              "Time stamp arr" <- w466
              n145 = feedback #1(u32 0) -> (w461:u32)
              n146 = Greater?(x=w460, y=w461) -> (0:w457:bool)
              n147 = Add(x=u32 300 ("y"), y=w460) -> (x+y=w462:u32)
              n148 = feedback-in #1(w462) -> ()
              n149 = Get Queue Status(queue=w468, error in (no error)=w471) -> (queue out=w467:refnum<queue>, error out=w470:errorcluster, # elements in queue=→"# elements in RAM queue":i32)  [unwired: 1 in, 5 out]
              n150 = case shown="True" w457 {
                tunnel: w463 -> [_ w478]
                frame False {
                }
                frame True {
                  n151 = Index Array(array=w478, index (dim 0)=0 ("disabled index (col)")) -> (element=w480:u32[][])  [unwired: 2 in]
                  "Image" <- w480
                  n152 = disable-structure shown="SCMP==COMP, Default" {
                    disable-tunnel: w480 -> [w481 w482]
                    frame condition #0 (active) {
                      "Camera T Image wide" <- w481
                      "Camera T Image" <- w481
                    }
                    frame condition #1 {
                      "Image Cam" <- w482
                    }
                  }
                }
              }
              n153 = Bundle By Name(cluster=w477, "Time Stamp Array"=w466) -> (w476:T12)
              n154 = case shown="True" "Save to FITS?" {
                tunnel: w476 -> [_ w491]
                tunnel: w475 -> [_ w490]
                tunnel: w455 -> [_ w489]
                tunnel: [w483 w486] -> w473
                tunnel: w470 -> [w483 w485]
                tunnel: w463 -> [_ w484]
                frame False {
                }
                frame True {
                  n155 = call "SCMP - Write FITS File v2.vi"("FITS Header"=w491, "Andor"=w490, "Data"=w484, "error in"=w485, "Image #"=w489) -> ("FITS Path Out"=w487:path, "error out"=w486:errorcluster)  [unwired: 8 in, 1 out]
                  n156 = Equal To 0?(x=w489) -> (x = 0?=w488:bool)
                  n157 = case shown="True" w488 {
                    tunnel: w487 -> [_ w492]
                    frame False {
                    }
                    frame True {
                      "FITS Path Out" <- w492
                    }
                  }
                }
              }
              n158 = Increment(x=w455) -> (x+1=w456:i32)
              n159 = local read "Break"() -> (w454:bool)
              "Image display & SSD Saving" <- w455
            }
            n160 = local read "Break"() -> (w443:bool)
          }
          n161 = for {
            N: w417 -> [_]
            tunnel: w439 -> [w514]
            tunnel: w437 -> [w512]
            tunnel: w431 -> [w511]
            tunnel: w433 -> [w510]
            shift-right: [w502] -> w430
            shift-left: w429 -> [w509]
            tunnel: w427 -> [w515]
            tunnel: [w513] -> w438
            tunnel: w423 -> [w501]
            tunnel: w424 -> [w495]
            shift-right: [w493] -> w419
            shift-left: u32 0 ("Image transfering") -> [w494]
            stop <- w508 stop-if-true
            n162 = for {
              N: w510 -> [_]
              tunnel: w515 -> [w547]
              tunnel: w514 -> [w544]
              tunnel: [w530] -> w513
              tunnel: w512 -> [w543]
              tunnel: w511 -> [w542]
              shift-right: [w535] -> w507
              shift-left: w495 -> [w536]
              shift-right: [w534] -> w506
              shift-left: w495 -> [w537]
              shift-right: [w533] -> w505
              shift-left: w495 -> [w538]
              shift-right: [w532] -> w504
              shift-left: w495 -> [w539]
              shift-right: [w526] -> w503
              shift-left: w509 -> [w524]
              tunnel: [w523] -> w499 mode=indexing
              tunnel: [w519] -> w508
              shift-right: [w516] -> w493
              shift-left: w494 -> [w517]
              i -> [w525]
              stop <- w519 stop-if-true
              n163 = Dequeue Element(queue=w547, timeout in ms (-1)=T17 11000 ("timeout for deque loop"), error in (no error)=w524) -> (queue out=w546:refnum<queue>, element=w545:u64, timed out?=w521:bool, error out=w528:errorcluster)
              n164 = Increment(x=w517) -> (x+1=w516:u32)
              n165 = call "SCD - Process Low Level Camera Data Into Image.vi"("Pointer In"=w545, "Neo Info"=w542, "ByteData (U8)"=w544, "PixelData (U16)"=w543, "error in (no error)"=w528, "scmp demo pic"=TRUE) -> ("Image (I32)"=w531:u32[][], "Timestamp"=w523:timestamp, "error out"=w527:errorcluster)  [unwired: 7 in]
              n166 = Or(x=w521, y="user break") -> (x .or. y?=w519:bool)
              n167 = Quotient & Remainder(x=w525, y=4) -> (x-y*floor(x/y)=w540:i32)  [unwired: 1 out]
              n168 = Get Queue Status(queue=w546, error in (no error)=w527) -> (queue out=w530:refnum<queue>, error out=w526:errorcluster, # elements in queue=→"# elements in queue":i32)  [unwired: 1 in, 5 out]
              n169 = case shown="0, Default" w540 {
                tunnel: w539 -> [w551 w558 w564 w567]
                tunnel: w538 -> [w552 w559 w561 w570]
                tunnel: w537 -> [w553 w555 w565 w571]
                tunnel: w536 -> [w549 w556 w562 w568]
                tunnel: [w548 w556 w562 w568] -> w535
                tunnel: [w553 w554 w565 w571] -> w534
                tunnel: [w552 w559 w560 w570] -> w533
                tunnel: [w551 w558 w564 w566] -> w532
                tunnel: w531 -> [w550 w557 w563 w569]
                frame 0, Default {
                  n170 = Add(x=w549, y=w550) -> (x+y=w548:u32[][])
                }
                frame 1 {
                  n171 = Add(x=w555, y=w557) -> (x+y=w554:u32[][])
                }
                frame 2 {
                  n172 = Add(x=w561, y=w563) -> (x+y=w560:u32[][])
                }
                frame 3 {
                  n173 = Add(x=w567, y=w569) -> (x+y=w566:u32[][])
                }
              }
              "Image transfering" <- w517
            }
            "Break" <- w508
            n174 = Build Array(w507, w506, w505, w504) -> (w497:u32[][][])
            n175 = Array Subset(array=w499, length=4) -> (w496:timestamp[])  [unwired: 1 in]
            n176 = Bundle(w497, w496) -> (w498:cluster{u32[][][], timestamp[]})  [unwired: 1 in]
            n177 = Enqueue Element(queue=w501, element=w498, error in (no error)=w503) -> (error out=w502:errorcluster)  [unwired: 1 in, 2 out]
          }
          n178 = for "Loop which waits for and build up list of image pointers for processing" {
            N: w434 -> [_]
            tunnel: w441 -> [w579]
            tunnel: [w579] -> w440
            tunnel: w427 -> [w577]
            shift-right: [w576] -> w432
            shift-left: w442 -> [w581]
            i -> [w573]
            stop <- w575 stop-if-true
            n179 = Increment(x=w573) -> (x+1=→"Image Acq":i32)
            n180 = call <userlib>:"AT Wait Buffer A.vi"("error in (no error)"=w581, "Timeout"=T17 11000 ("timeout for deque loop"), "Handle"=w579) -> ("error out"=w578:errorcluster, "Output buffer"=w580:u64)  [unwired: 5 in, 2 out]
            n181 = case shown="No Error" w578 {
              selector: w578 -> [w583 w592]
              tunnel: w580 -> [w585 _]
              tunnel: [w582 w592] -> w576
              tunnel: w577 -> [w584 _]
              frame No Error {
                n182 = local read "image pointers"() -> (w589:u64[])
                n183 = Enqueue Element(queue=w584, element=w585, error in (no error)=w583) -> (error out=w582:errorcluster)  [unwired: 1 in, 2 out]
                n184 = local read "count"() -> (w591:i32)
                n185 = local read "imageNo"() -> (w586:i32)
                n186 = Increment(x=w591) -> (x+1=w590:i32)
                n187 = Insert Into Array(array=w589, index=w586, new element=w585) -> (w588:u64[])
                n188 = Increment(x=w586) -> (x+1=w587:i32)
                n189 = local write "count"(w590) -> ()
                n190 = local write "imageNo"(w587) -> ()
                n191 = local write "image pointers"(w588) -> ()
              }
              frame Error {
              }
            }
            n192 = local read "Break"() -> (w575:bool)
          }
          n193 = local write "Image transfering"(w419) -> ()
          n194 = local write "Image display & SSD Saving"(w420) -> ()
          n195 = disable-structure shown="Disabled" {
            frame Disabled {
              n196 = call "SCMP - picture flip rotate.vi"() -> ()  [unwired: 8 in, 4 out]
            }
            frame Enabled {
            }
          }
        }
        frame #1 {
          n197 = call <userlib>:"AT Command A.vi"("Feature"="AcquisitionStop" ("Command"), "Handle"=w596) -> ()  [unwired: 8 in, 2 out]
        }
        frame #2 {
          n198 = call <userlib>:"AT Flush A.vi"("Handle"=w604) -> ()  [unwired: 9 in, 2 out]
          n199 = call <userlib>:"AT Clear All Buffers A.vi"("Handle"=w604) -> ("error out"=w603:errorcluster)  [unwired: 9 in, 1 out]
          n200 = Merge Errors(w603, w605) -> (w606:errorcluster)
        }
      }
      n201 = call "SCD - Timestamp AO Waveform.vi"("DAQ To"=w79, "SCD AO Waveforms"=w104) -> ()  [unwired: 8 in, 2 out]
      n202 = call <vilib>:"DAQmx Start Task.vi"("task/channels in"=w74, "error in"=w117) -> ("task out"=w140:refnum<k21>, "error out"=w57:errorcluster)  [unwired: 12 in]
      n203 = call "PDSS - Turn Trigger Light On.vi"("error in (no error)"=w57) -> ("error out"=w132:errorcluster, "Trigger Started"=→"Image Acquisition Started":bool)  [unwired: 9 in]
      n204 = Multiply(x=1000.0, y=w22) -> (x*y=w58:dbl)
      n205 = disable-structure shown="Disabled" {
        disable-tunnel: w140 -> [w153 w155]
        disable-tunnel: w132 -> [w152 w154]
        disable-tunnel: [w150 w154] -> w24
        disable-tunnel: w22 -> [w148 _]
        disable-tunnel: [_ w155] -> w21
        frame Disabled {
          n206 = Multiply(x=w148, y=1.25 ("x")) -> (x*y=w151:dbl)
          n207 = call <vilib>:"DAQmx Wait Until Done.vi"("task/channels in"=w153, "timeout (sec)"=w151, "error in"=w152) -> ("error out"=w150:errorcluster)  [unwired: 11 in, 1 out]
        }
        frame Enabled {
        }
      }
      n208 = property on="Image Acq (s)" class="Slide (strict)"(error in=w57, "Scale.Maximum"=w58) -> (error out=w56:errorcluster)  [unwired: 1 in, 1 out]
      n209 = while {
        tunnel: w58 -> [w171]
        tunnel: w56 -> [_]
        tunnel: w24 -> [w178]
        tunnel: [w177] -> w23
        tunnel: w21 -> [w176]
        tunnel: [w175] -> w20
        tunnel: [w170] -> w18
        i -> [w180]
        stop <- w174 stop-if-true
        w179 = u32 300 ("milliseconds to wait")
        n210 = Multiply(x=w180, y=w179) -> (x*y=w181:u32)
        n211 = Wait (ms)(milliseconds to wait=w179) -> ()  [unwired: 1 out]
        n212 = Subtract(x=w171, y=w181) -> (x-y=w170:dbl)
        "Image Acq (s)" <- w170
        n213 = call <vilib>:"DAQmx Is Task Done.vi"("task/channels in"=w176, "error in"=w178) -> ("task out"=w175:refnum<k21>, "task done?"=w173:bool, "error out"=w177:errorcluster)  [unwired: 11 in]
        n214 = local read "Break"() -> (w172:bool)
        n215 = Or(x=w172, y=w173) -> (x .or. y?=w174:bool)
      }
      n216 = Multiply(x=w18, y=0.0 ("Image Acq (s)")) -> (x*y=w17:dbl)
      n217 = call <vilib>:"DAQmx Stop Task.vi"("task/channels in"=w20, "error in"=w23) -> ("task out"=w139:refnum<k21>, "error out"=w138:errorcluster)  [unwired: 12 in]
      n218 = local write "Image Acq (s)"(w17) -> ()
      n219 = call <vilib>:"DAQmx Clear Task.vi"("task in"=w139, "error in"=w138) -> ("error out"=w127:errorcluster)  [unwired: 13 in]
      n220 = invoke on="Image Acquisition Started" class="Bool (strict)" method="Reinit To Default"(error in=w127) -> (error out=w126:errorcluster)  [unwired: 2 in, 2 out]
      n221 = disable-structure shown="SCMP==SCD" {
        disable-tunnel: [tag "PXI-6733/port0/line0" ("lines") tag "Dev3/port0/line0" ("comp lines")] -> w101
        disable-tunnel: [tag "PXI-6733/ao0:7" ("physical channels") tag "Dev3/ao0:7" ("physical channels")] -> w100
        frame condition #0 {
        }
        frame condition #1 (active) {
        }
      }
      n222 = call "SCD - Trigger Sequence - Set All AO Values to Zero.vi"("error in"=w126, "lines"=w101, "physical channels"=w100) -> ("error out"=w121:errorcluster)  [unwired: 8 in]
      n223 = global read "Global demo.vi" "demo"() -> (w15:bool)
      n224 = Release Queue(queue=w44, error in (no error)=w42) -> (error out=w43:errorcluster)  [unwired: 1 in, 2 out]
      n225 = Release Queue(queue=w108, error in (no error)=w107) -> (error out=w103:errorcluster)  [unwired: 1 in, 2 out]
      n226 = Merge Errors(w68, w103, w76, w43) -> (w19:errorcluster)
      n227 = case shown="True" w15 {
        tunnel: w19 -> [_ w147]
        frame False {
        }
        frame True {
          # "len ukoncenie daq slucky\n v demo mode skor"
          n228 = property on="Break" class="Bool (strict)"(error in=w147, "Value"=TRUE ("Break")) -> ()  [unwired: 1 in, 2 out]
        }
      }
      n229 = Merge Errors(w19, w121) -> (w120:errorcluster)
      "Headers Out" <- w106
      "error cam dequeue & queue RAM" <- w76
      "Time Start" <- w79
      "error dequeue RAM" <- w42
    }
    frame Error {
    }
  }
  "error out" <- w9
  n230 = disable-structure shown="Disabled" {
    frame Disabled {
      # "someday this\nmight speed up\naccumulatons"
      n231 = call "SCD - Extract Image Vector and Timestamp from Pointer.vi"() -> ()  [unwired: 13 in, 3 out]
    }
    frame Enabled {
    }
  }
